vi "Replicate Core.vi"(9 "# event structures":u16=2, 10 "msg (unused)":cluster{"cmd":string, "data":variant}, 11 "data in":refnum<class "EventMessengerPData.lvclass">) -> (2 "Event Registration Refnum":refnum<event-registration>[](array[refnum]), 3 "data out":refnum<class "EventMessengerPData.lvclass">)   [LabVIEW 2020, in "Event Messenger Priority.lvlib" / "EventMessengerPData.lvclass"]
uses:
  EventMessengerPData.lvclass
  EventMessengerPData.lvclass/EventMessengerPData.ctl
  Event Data.ctl
  Event Messenger Priority.lvlib
  Element.ctl
panel:
  # "See note on block diagram."
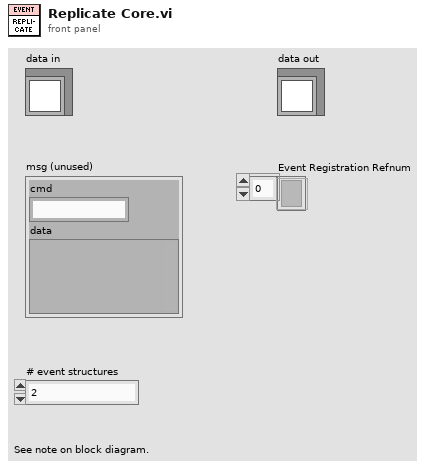
[diagram p1: front panel]
types:
  T1 = typedef "Event Messenger Priority.lvlib/Event Data.ctl" = cluster{"elt":T2, "elt valid?":bool, "last elt?":bool, "aborted?":bool, "priority?":bool}
  T2 = typedef "Event Messenger Priority.lvlib/Element.ctl" = cluster{"cmd":string, "data":variant}
  T3 = typedef "Custom Event Messenger.lvlib/Element.ctl" = cluster{"cmd":string, "data":variant}
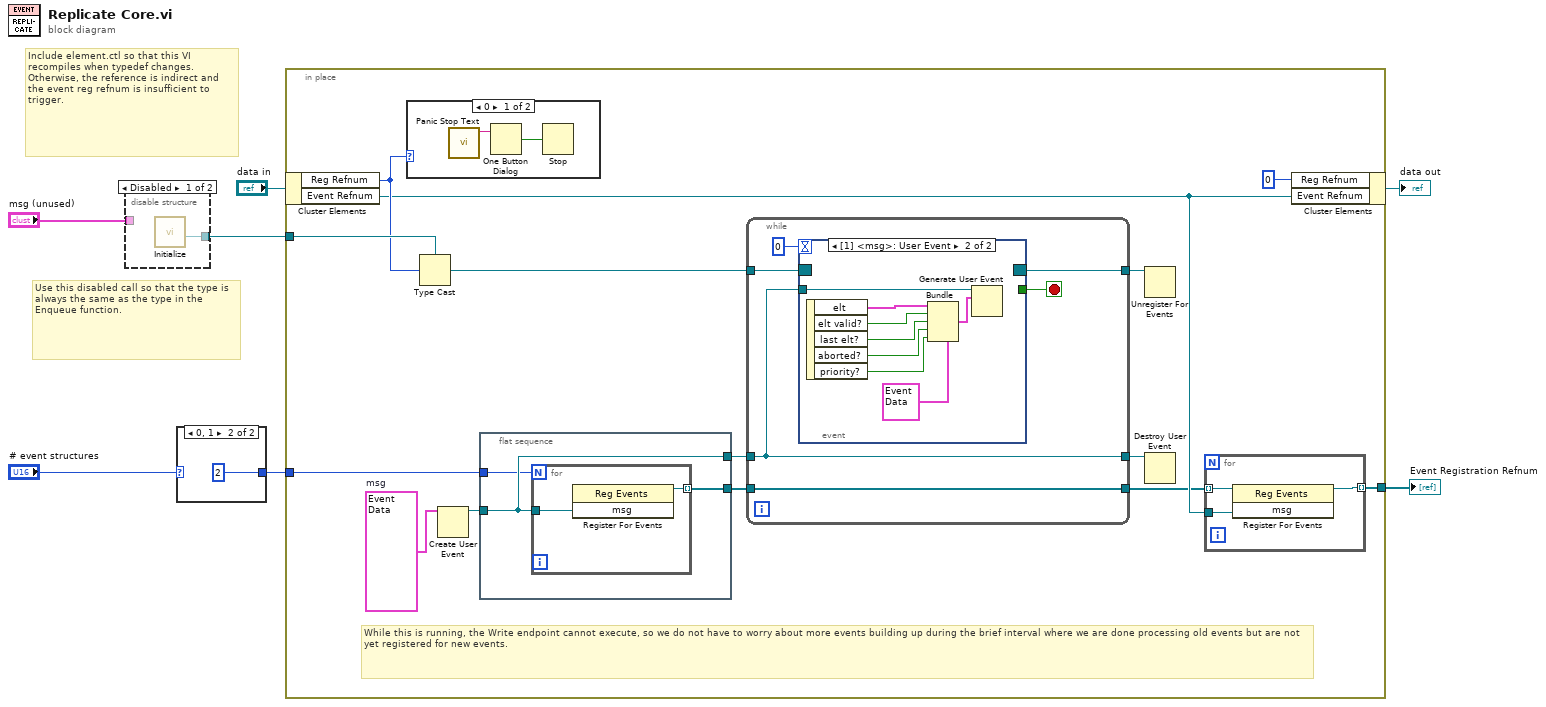
[diagram p0: block diagram]
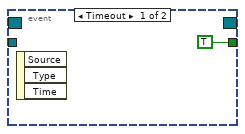
[diagram p4: hidden frame]
diagram:
  # "Include element.ctl so that this VI recompiles when typedef changes. Otherwise, the reference is indirect and the event reg refnum is insufficient to trigger."
  # "Use this disabled call so that the type is always the same as the type in the Enqueue function."
  n1 = disable-structure shown="Disabled" {
    disable-tunnel: [w8 _] -> w7
    disable-tunnel: "msg (unused)" -> [_ _]
    frame Disabled {
      n2 = call "Initialize.vi"() -> ("Event Registration Refnum"=w8:refnum<event-registration>)  [unwired: 10 in, 1 out]
    }
    frame Enabled {
    }
  }
  n3 = case shown="0, 1" "# event structures" {
    selector: "# event structures" -> [w9 _]
    tunnel: [w9 u16 2] -> w3
    frame Default {
    }
    frame 0, 1 {
    }
  }
  n4 = in-place {
    in-place-border: w7 -> [w24]
    in-place-border: w3 -> [w15]
    in-place-border: [w11] -> w2
    w12 = T1 {"elt"={"cmd"="", "data"=variant(bool FALSE)}, "elt valid?"=TRUE, "last elt?"=FALSE, "aborted?"=FALSE, "priority?"=FALSE}  # msg
    # "While this is running, the Write endpoint cannot execute, so we do not have to worry about more events building up during the brief interval where we are done processing old events but are not yet registered for new events."
    n5 = in-place-cluster #1("data in") -> ("Reg Refnum"=w22:u32, "Event Refnum"=w20:refnum<user-event>)
    n6 = case shown="0" w22 {
      frame 0 {
        n7 = call "Panic Stop Text.vi"() -> ("Text"=w48:string)  [unwired: 11 in]
        n8 = One Button Dialog(message=w48) -> (true=w49:bool)  [unwired: 1 in]
        n9 = Stop(stop? (T)=w49) -> ()
      }
      frame Default {
      }
    }
    n10 = Type Cast(type=w24, x=w22) -> (*(type *) &x=w21:refnum<event-registration>)
    n11 = Create User Event(user event datatype=w12) -> (user event=w17:refnum<user-event>)  [unwired: 1 in, 1 out]
    n12 = flat-sequence {
      tunnel: [w27] -> w19
      tunnel: w17 -> [w26]
      tunnel: [w26] -> w16
      tunnel: w15 -> [w25]
      frame #0 {
        n13 = for {
          N: w25 -> [_]
          tunnel: w26 -> [w29]
          tunnel: [w28] -> w27 mode=indexing
          n14 = register-events(w29) -> (reference out=w28:refnum<event-registration>)  [unwired: 2 in, 1 out]
        }
      }
    }
    n15 = while {
      tunnel: w21 -> [w38]
      tunnel: [w35] -> w18
      tunnel: w19 -> [w35]
      tunnel: w16 -> [w34]
      tunnel: [w34] -> w14
      tunnel: [w33] -> w13
      stop <- w36 stop-if-true
      n16 = event shown="[1] <msg>: User Event" {
        selector: w38 -> [_ _]
        dyn-events: [_ _] -> w33
        timeout: 0 -> [_ _]
        tunnel: [TRUE _] -> w36
        tunnel: w34 -> [_ w47]
        event Timeout {
          n17 = event-data() -> ()  [unwired: 1 in, 3 out]
        }
        event User Event {
          n18 = event-data() -> ("elt"=w46:T3, "elt valid?"=w45:bool, "last elt?"=w44:bool, "aborted?"=w43:bool, "priority?"=w41:bool)  [unwired: 1 in]
          n19 = Bundle(cluster=T1 {"elt"={"cmd"="", "data"=variant}, "elt valid?"=TRUE, "last elt?"=TRUE, "aborted?"=TRUE, "priority?"=TRUE} ("msg"), "elt"=w46, "elt valid?"=w45, "last elt?"=w44, "aborted?"=w43, "priority?"=w41) -> (w42:T1)
          n20 = Generate User Event(user event=w47, event data cluster=w42) -> ()  [unwired: 2 in, 2 out]
        }
      }
    }
    n21 = Unregister For Events(event registration refnum=w13) -> ()  [unwired: 1 in, 1 out]
    n22 = Destroy User Event(user event=w14) -> ()  [unwired: 1 in, 1 out]
    n23 = for {
      tunnel: w20 -> [w32]
      tunnel: w18 -> [w31] mode=indexing
      tunnel: [w30] -> w11 mode=indexing
      n24 = register-events(reference=w31, w32) -> (reference out=w30:refnum<event-registration>)  [unwired: 1 in, 1 out]
    }
    n25 = in-place-cluster #1("Reg Refnum"=u32 0, "Event Refnum"=w20) -> (→"data out":refnum<class "EventMessengerPData.lvclass">)
  }
  "Event Registration Refnum" <- w2
